vi "Log Values Example.vi"() -> ()   [LabVIEW 2017, in "Logger Examples.lvlib"]
uses:
  <vilib>/gpm_packages/@cs/event-logger/Examples/Logger Examples.lvlib
  <vilib>/gpm_packages/@cs/event-logger/Source/Composed Log/Types/Log Level.ctl
  <vilib>/gpm_packages/@cs/event-logger/Source/HTML File Sink/HTML File Format.lvclass
  C:/Program Files/National Instruments/LabVIEW 2017/vi.lib/gpm_packages/@cs/event-logger/Source/IStringFormat/IStringFormat.lvclass
  <vilib>/gpm_packages/@cs/event-logger/Source/String Formats/String Expression Format/String Expression Format.lvclass/String Expression Format.ctl
  <vilib>/gpm_packages/@cs/event-logger/Source/Composed Log/LoggerReference/LoggerReference.lvclass/LoggerReference.ctl
  cb6cc8f4-355e-4f60-beee-1dac019a5190.vi
  d053d638-c5ca-4061-b75c-930c5d54a4a0.vi
  a4aecb2a-c8ab-40e1-948d-3fbd1094d214.vi
  d9747495-8d6c-4d86-9b58-ec7b36ea6678.vi
  13ff8fb6-9e5d-4405-b0df-27c05d5aea20.vi
  9f234408-1270-49d7-b342-8c2f3c962d83.vi
  150d9d2d-db35-4e36-bc8e-367fbd223884.vi
  57f424a8-0347-4995-a908-3cdd2378fbfa.vi
  261ea4dc-86e2-4e22-a46e-fc1e124681f7.vi
  <vilib>/gpm_packages/@cs/event-logger/Source/String Formats/String Expression Format/Run Formatter.vi
  <vilib>/gpm_packages/@cs/event-logger/Source/Composed Log/LoggerReference/Return Aggregate Queues.vi
  <vilib>/gpm_packages/@cs/event-logger/Source/Composed Log/LoggerReference/Add Aggregate Log.vi
  cb6cc8f4-355e-4f60-beee-1dac019a5190.vi/f0589759-63da-4caa-be49-6820fd9972fe.vi
  a4aecb2a-c8ab-40e1-948d-3fbd1094d214.vi/3efe23c9-ad5f-4d29-af96-d54db191a5d3.vi
  <vilib>/gpm_packages/@cs/event-logger/Source/Composed Log/LoggerReference/Get Valid Event Time.vi
  <vilib>/gpm_packages/@cs/event-logger/Source/Composed Log/LoggerReference/Log Event.vi
  d9747495-8d6c-4d86-9b58-ec7b36ea6678.vi/2c9614b8-4e16-454c-b74d-0797d092026b.vi
  13ff8fb6-9e5d-4405-b0df-27c05d5aea20.vi/c7b07c83-97a3-4976-a25c-8cfc57cdcc99.vi
  9f234408-1270-49d7-b342-8c2f3c962d83.vi/74885dca-9492-4c3c-b816-4c26e2ec6fcd.vi
  150d9d2d-db35-4e36-bc8e-367fbd223884.vi/f3cfdab1-a8d5-4285-8046-bdf2d6b5393d.vi
  57f424a8-0347-4995-a908-3cdd2378fbfa.vi/ee3f39dd-221c-44f5-8768-2f297b0c434c.vi
  <vilib>/gpm_packages/@cs/event-logger/Source/Composed Log/LoggerReference/Get Formatter.vi
  261ea4dc-86e2-4e22-a46e-fc1e124681f7.vi/cd1d683c-0b51-4f8f-9779-dd35a2ed2214.vi
  <vilib>/dlg_ctls.llb/Space Constant.vi
  <vilib>/gpm_packages/@cs/event-logger/Source/Composed Log/LoggerReference/Send Add Sink.vi
  <vilib>/gpm_packages/@cs/event-logger/Source/Composed Log/LoggerReference/Log.vi
  <vilib>/gpm_packages/@cs/event-logger/Source/Composed Log/LoggerReference/Remove Stale Logs.vi
  <vilib>/gpm_packages/@cs/event-logger/Source/String Control Sink/String Control Sink.lvclass
  C:/Program Files/National Instruments/LabVIEW 2017/vi.lib/gpm_packages/@cs/event-logger/Source/Composed Log/Log Sink/Log Sink.lvclass
  <vilib>/gpm_packages/@cs/event-logger/Source/Composed Log/Application Logger/Launch Worker Loop.vi
  <vilib>/gpm_packages/@cs/event-logger/Source/Composed Log/LoggerReference/Initialize Logger Instance.vi
  <vilib>/gpm_packages/@cs/event-logger/Source/Composed Log/LoggerReference/Format Variant.vi
  <vilib>/gpm_packages/@cs/event-logger/Source/String Formats/String Expression Format/String Expression Format.lvclass
  <vilib>/gpm_packages/@cs/event-logger/Source/Composed Log/LoggerReference/LoggerReference.lvclass
  <vilib>/gpm_packages/@cs/event-logger/Source/Composed Log/IErrorFormat/IErrorFormat.lvclass
  <vilib>/gpm_packages/@cs/event-logger/Source/Composed Log/Log Sink/Log Sink.lvclass
  <vilib>/gpm_packages/@cs/event-logger/Examples/GenericSerializable/GenericSerializable.lvclass
  <vilib>/gpm_packages/@cs/event-logger/Source/Composed Log/Composed Log.lvlib
panel:
  out "Event Log":string
  # "Run the VI, then view the block diagram notes for details on formatting various data types."
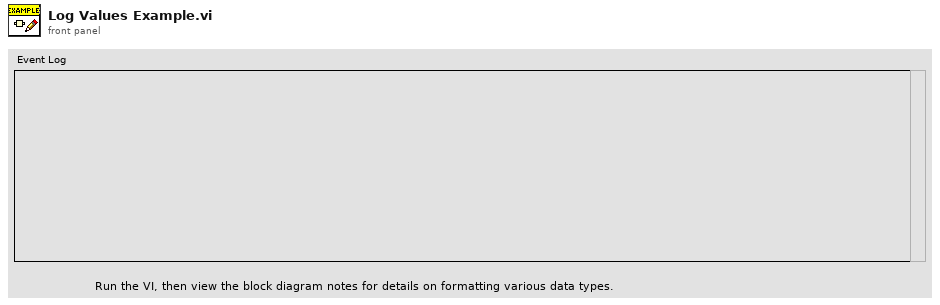
[diagram p1: front panel]
types:
  T1 = typedef "Composed Log.lvlib/Log Level.ctl" = enum16{"Debug", "Info", "Warning", "Error", "Critical"}
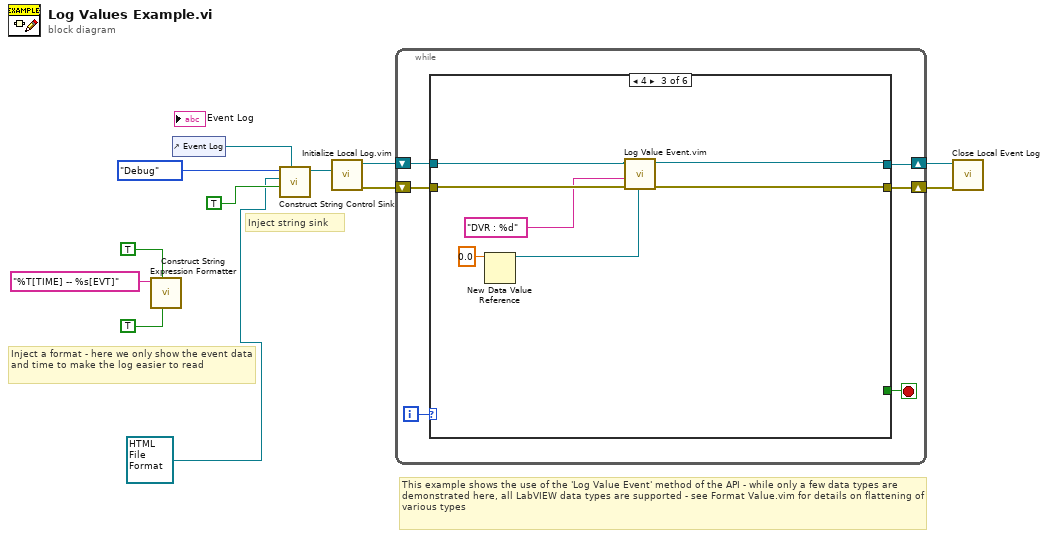
[diagram p0: block diagram]
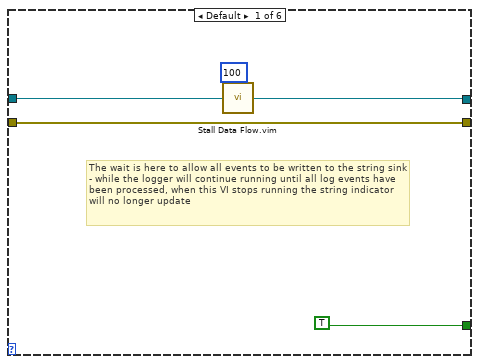
[diagram p2: hidden frame]
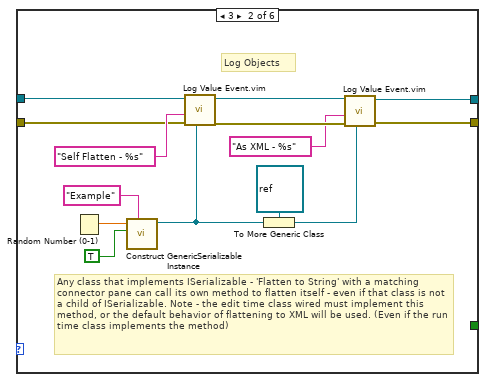
[diagram p3: hidden frame]
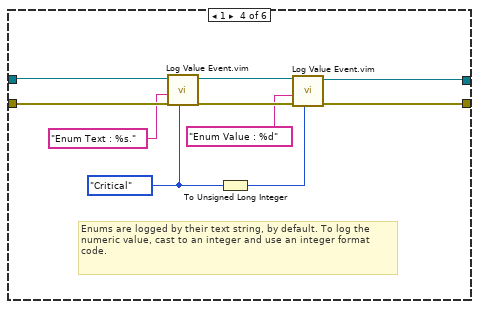
[diagram p4: hidden frame]
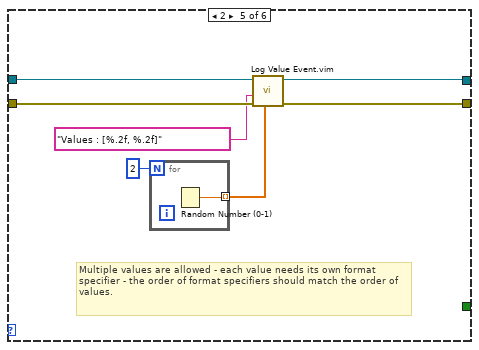
[diagram p5: hidden frame]
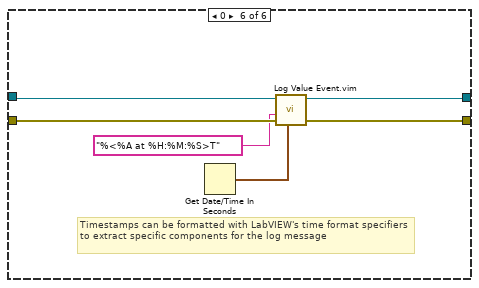
[diagram p6: hidden frame]
diagram:
  # "This example shows the use of the 'Log Value Event' method of the API - while only a few data types are demonstrated here, all LabVIEW data types are supported - see Format Value.vim for details on flattening of various types"
  # "Inject string sink"
  # "Inject a format - here we only show the event data and time to make the log easier to read"
  n1 = call <vilib>:"Construct String Expression Formatter.vi"("Remove LineFeeds?(F)"=TRUE, "Append EOL?"=TRUE, "Format Specifier"="%T[TIME] -- %s[EVT]") -> ()  [unwired: 7 in, 2 out]
  n2 = control-ref of="Event Log"() -> (w11:refnum<vi>)
  n3 = call <vilib>:"Construct String Control Sink.vi"("Str Refnum"=w11, "AutoScroll?(F)"=TRUE, "LogFormat"=refnum<class "HTML File Format.lvclass"> refnum ("HTML File Format.lvclass"), "LogLevel"=Log_Level."Debug") -> ("String Control Sink out"=w2:refnum<class "String Control Sink.lvclass">)  [unwired: 7 in]
  n4 = call "Initialize Local Log.vim"("Startup Sink(s)"=w2) -> ("error out"=w6:errorcluster, "Log Instance Reference"=w5:refnum<class "LoggerReference.lvclass">)  [unwired: 8 in, 1 out]
  n5 = while {
    shift-right: [w15] -> w3
    shift-left: w6 -> [w18]
    shift-right: [w16] -> w4
    shift-left: w5 -> [w17]
    i -> [w14]
    stop <- w13 stop-if-true
    n6 = case shown="4" w14 {
      tunnel: w18 -> [w23 w26 w42 w51 w57 w65]
      tunnel: w17 -> [w20 w27 w43 w52 w58 w66]
      tunnel: [w19 w31 w38 w53 w59 w68] -> w16
      tunnel: [w23 w30 w39 w54 w60 w67] -> w15
      tunnel: [TRUE _ _ _ _ _] -> w13
      frame Default {
        # "The wait is here to allow all events to be written to the string sink - while the logger will continue running until all log events have been processed, when this VI stops running the string indicator will no longer update"
        n7 = call "Stall Data Flow.vim"("value in"=w20, "milliseconds to wait"=u32 100) -> ("value out"=w19:refnum<class "LoggerReference.lvclass">)  [unwired: 1 out]
      }
      frame 3 {
        # "Log Objects"
        # "Any class that implements ISerializable - 'Flatten to String' with a matching connector pane can call its own method to flatten itself - even if that class is not a child of ISerializable. Note - the edit time class wired must implement this method, or the default behavior of flattening to XML will be used. (Even if the run time class implements the method)"
        n8 = Random Number (0-1)() -> (number: 0 to 1=w35:dbl)
        n9 = call <vilib>:"Construct GenericSerializable Instance.vi"("InstanceID"="Example", "Boolean Data"=TRUE, "Numeric Data"=w35) -> ("GenericSerializable out"=w25:refnum<class "GenericSerializable.lvclass">)  [unwired: 8 in]
        n10 = call "Log Value Event.vim"("Value(s)"=w25, "error in (no error)"=w26, "Log Message Format String"="Self Flatten - %s" ("Log Message"), "LoggerReference in"=w27) -> ("error out"=w32:errorcluster, "LoggerReference out"=w33:refnum<class "LoggerReference.lvclass">)  [unwired: 6 in]
        n11 = To More Generic Class(target class=refnum<class> refnum ("LabVIEW Object"), reference=w25) -> (generic class reference=w24:refnum<class>)
        n12 = call "Log Value Event.vim"("Value(s)"=w24, "error in (no error)"=w32, "Log Message Format String"="As XML - %s" ("Log Message"), "LoggerReference in"=w33) -> ("error out"=w30:errorcluster, "LoggerReference out"=w31:refnum<class "LoggerReference.lvclass">)  [unwired: 6 in]
      }
      frame 4 {
        n13 = New Data Value Reference(data value=0.0) -> (data value reference=w41:refnum<data-value>)  [unwired: 1 in, 1 out]
        n14 = call "Log Value Event.vim"("Value(s)"=w41, "error in (no error)"=w42, "Log Message Format String"="DVR : %d", "LoggerReference in"=w43) -> ("error out"=w39:errorcluster, "LoggerReference out"=w38:refnum<class "LoggerReference.lvclass">)  [unwired: 6 in]
      }
      frame 1 {
        w46 = Log_Level."Critical" ("Event Level")
        # "Enums are logged by their text string, by default. To log the numeric value, cast to an integer and use an integer format code."
        n15 = call "Log Value Event.vim"("Value(s)"=w46, "error in (no error)"=w51, "Log Message Format String"="Enum Text : %s." ("Log Message"), "LoggerReference in"=w52) -> ("error out"=w49:errorcluster, "LoggerReference out"=w50:refnum<class "LoggerReference.lvclass">)  [unwired: 6 in]
        n16 = To Unsigned Long Integer(number=w46) -> (unsigned 32bit integer=w45:u32)
        n17 = call "Log Value Event.vim"("Value(s)"=w45, "error in (no error)"=w49, "Log Message Format String"="Enum Value : %d" ("Log Message"), "LoggerReference in"=w50) -> ("error out"=w54:errorcluster, "LoggerReference out"=w53:refnum<class "LoggerReference.lvclass">)  [unwired: 6 in]
      }
      frame 2 {
        # "Multiple values are allowed - each value needs its own format specifier - the order of format specifiers should match the order of values."
        n18 = for {
          N: 2 -> [_]
          tunnel: [w62] -> w55 mode=indexing
          n19 = Random Number (0-1)() -> (number: 0 to 1=w62:dbl)
        }
        n20 = call "Log Value Event.vim"("Value(s)"=w55, "error in (no error)"=w57, "Log Message Format String"="Values : [%.2f, %.2f]" ("Log Message"), "LoggerReference in"=w58) -> ("error out"=w60:errorcluster, "LoggerReference out"=w59:refnum<class "LoggerReference.lvclass">)  [unwired: 6 in]
      }
      frame 0 {
        # "Timestamps can be formatted with LabVIEW's time format specifiers to extract specific components for the log message"
        n21 = Get Date/Time In Seconds() -> (seconds since 1Jan1904=w64:timestamp)
        n22 = call "Log Value Event.vim"("Value(s)"=w64, "error in (no error)"=w65, "Log Message Format String"="%<%A at %H:%M:%S>T", "LoggerReference in"=w66) -> ("error out"=w67:errorcluster, "LoggerReference out"=w68:refnum<class "LoggerReference.lvclass">)  [unwired: 6 in]
      }
    }
  }
  n23 = call <vilib>:"Close Local Event Log.vi"("error in (no error)"=w3, "Log Instance"=w4) -> ()  [unwired: 9 in, 1 out]
